vi "Get Block Diagram Image Sizes.vi"(8 "Error In":errorcluster, 10 "Images Directory":path, 11 "Image Names":string[](array[string])) -> (0 "Error Out":errorcluster, 3 "Block Diagram Images":T1[](array[typedef]))   [LabVIEW 2014, in "i3-docs.lvlib"]
uses:
  i3-docs.lvlib
  Controls/image_information.ctl
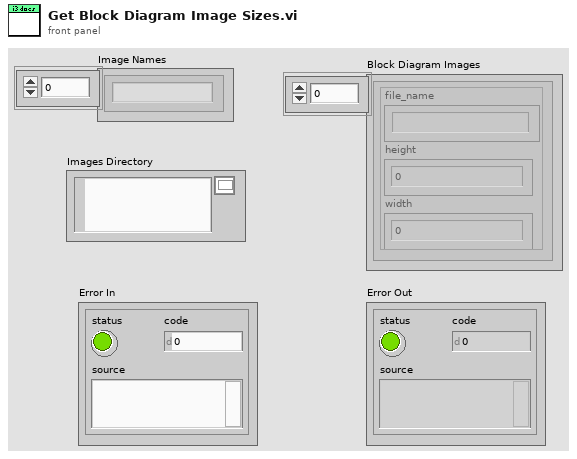
[diagram p1: front panel]
types:
  T1 = typedef "i3-docs.lvlib/image_information.ctl" = cluster{"file_name":string, "height":i32, "width":i32}
  T2 = typedef "imagedata.ctl" = cluster{"image type":i32, "image depth":i32, "image":u8[], "mask":u8[], "colors":u32[], "Rectangle":cluster{"left":i16, "top":i16, "right":i16, "bottom":i16}}
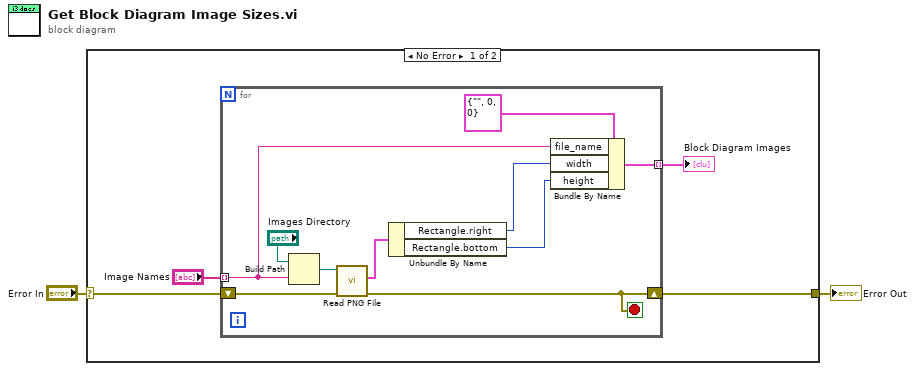
[diagram p0: block diagram]
diagram:
  n1 = case shown="No Error" "Error In" {
    selector: "Error In" -> [w5 w17]
    tunnel: [w4 w17] -> w1
    frame No Error {
      n2 = for {
        tunnel: "Image Names" -> [w9] mode=indexing
        shift-right: [w7] -> w4
        shift-left: w5 -> [w14]
        tunnel: [w8] -> w3 mode=indexing
        stop <- w7 stop-if-true
        n3 = Build Path(base path="Images Directory", name or relative path=w9) -> (appended path=w15:path)
        n4 = call <vilib>:"Read PNG File.vi"("error in (no error)"=w14, "path to PNG file"=w15) -> ("error out"=w7:errorcluster, "image data"=w13:T2)  [unwired: 7 in, 1 out]
        n5 = Unbundle By Name(w13) -> ("Rectangle.right"=w11:i16, "Rectangle.bottom"=w10:i16)
        n6 = Bundle By Name(cluster=T1 {"file_name"="", "height"=0, "width"=0} ("block_diagram_image"), "file_name"=w9, "width"=w11, "height"=w10) -> (w8:T1)
      }
      "Block Diagram Images" <- w3
    }
    frame Error {
    }
  }
  "Error Out" <- w1
